vi "GetEvents.vi"(8 "error in (no error)":errorcluster, 11 "Tree View in":refnum<class "FastTreeView.lvclass">) -> (0 "error out":errorcluster, 2 "CellClicked":refnum<user-event>, 3 "Tree View out":refnum<class "FastTreeView.lvclass">)   [LabVIEW 2025, in "FastTreeView.lvclass"]
uses:
  FastTreeView.lvclass
  FastTreeView.lvclass/FastTreeView.ctl
  CellClicked--callback.vi
  C:/Git/FastTreeView/FastTreeView/LV/FastTreeView/dll/FastTreeView.dll
  dll/FastTreeView.dll
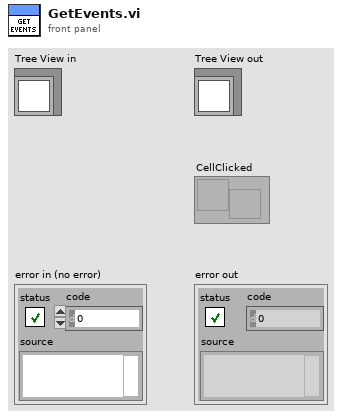
[diagram p1: front panel]
types:
  T1 = cluster{"Column":i32, "Tag":string, "IsExpander":bool, "IsGlyph":bool}
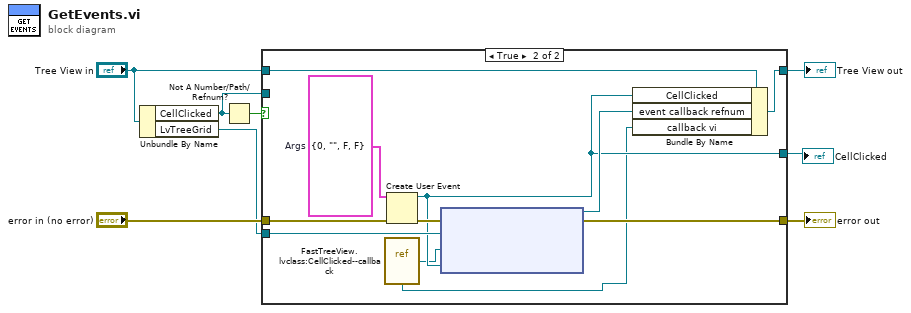
[diagram p0: block diagram]
diagram:
  n1 = Unbundle By Name("Tree View in") -> ("CellClicked"=w1:refnum<user-event>, "LvTreeGrid"=w3:refnum<k24>)
  n2 = Not A Number/Path/Refnum?(number/path/refnum=w1) -> (NaN/Path/Refnum?=w4:bool)
  n3 = case shown="True" w4 {
    tunnel: w3 -> [_ w20]
    tunnel: [w11 w19] -> w7
    tunnel: "error in (no error)" -> [w11 w18]
    tunnel: "Tree View in" -> [w10 w16]
    tunnel: [w10 w14] -> w5
    tunnel: [w9 w13] -> w2
    tunnel: w1 -> [w9 _]
    frame False {
    }
    frame True {
      w21 = T1 {"Column"=0, "Tag"="", "IsExpander"=FALSE, "IsGlyph"=FALSE}  # Args
      n4 = vi-ref "FastTreeView.lvclass:CellClicked--callback.vi"() -> ("vi reference"=w12:refnum<vi>)
      n5 = Create User Event(user event datatype=w21, error in=w18) -> (user event=w13:refnum<user-event>, error out=w17:errorcluster)
      n6 = node(w17, w20, w12, w13) -> (w15:refnum<k27>, w19:errorcluster)  [unwired: 1 in]
      n7 = Bundle By Name(cluster=w16, "CellClicked"=w13, "event callback refnum"=w15, "callback vi"=w12) -> (w14:refnum<class "FastTreeView.lvclass">)
    }
  }
  "error out" <- w7
  "Tree View out" <- w5
  "CellClicked" <- w2
